vi "dash safety data.vi"(2 "Mechanism":enum16{"Drive Train"}(ring), 5 "Menu":T1) -> ()   [LabVIEW 2014]
uses:
  typedefs/fg_getset.ctl
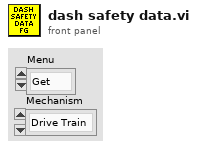
[diagram p1: front panel]
types:
  T1 = typedef "fg_getset.ctl" = enum16{"Get", "Set"}
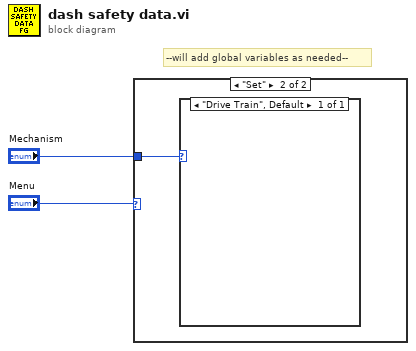
[diagram p0: block diagram]
diagram:
  # "--will add global variables as needed--"
  n1 = case shown="\"Set\"" "Menu" {
    tunnel: "Mechanism" -> [_ w3]
    frame "Get", Default {
    }
    frame "Set" {
      n2 = case shown="\"Drive Train\", Default" w3 {
        frame "Drive Train", Default {
        }
      }
    }
  }
